vi "Begin.vi"(8 "error in (no error)":errorcluster, 11 "Receiver in":refnum<class "Receiver.lvclass">) -> (0 "error out":errorcluster, 3 "Receiver out":refnum<class "Receiver.lvclass">)   [LabVIEW 2013, in "Receiver.lvlib" / "Receiver.lvclass"]
uses:
  Receiver.lvclass
  Receiver.lvclass/Receiver.ctl
  System/System.lvclass
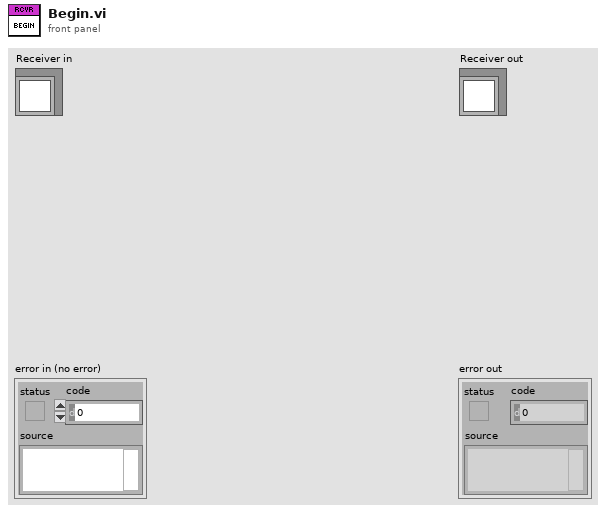
[diagram p1: front panel]
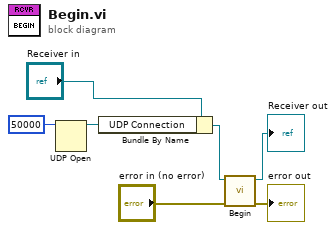
[diagram p0: block diagram]
diagram:
  n1 = UDP Open(11:u16 50000 ("port")) -> (port=w1:refnum<k16>)  [unwired: 4 in, 2 out]
  n2 = Bundle By Name(cluster="Receiver in", "UDP Connection"=w1) -> (w2:refnum<class "Receiver.lvclass">)
  n3 = call-parent "Begin.vi"("error in (no error)"="error in (no error)", "System in"=w2) -> ("error out"=→"error out":errorcluster, "System out"=→"Receiver out":refnum<class "Receiver.lvclass">)  [unwired: 8 in]
